vi "PRAMMS-DataString2Image.vi"(7 "ImageData":u8[](array[numeric])) -> (1 "Width":u16, 2 "Height":u16, 3 "BitPerPixel":u32, 8 "Image":u16[][](array[numeric]), 12 "TimeStamp?":u64, 13 "ImageID":u32, 14 "ImageFrameRate":dbl format="%.2f")   [LabVIEW 2019]
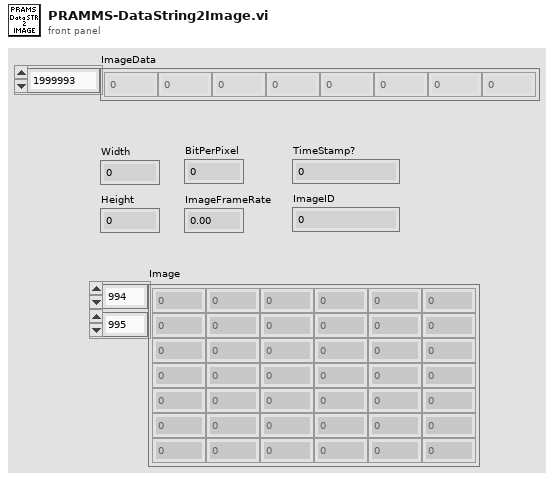
[diagram p1: front panel]
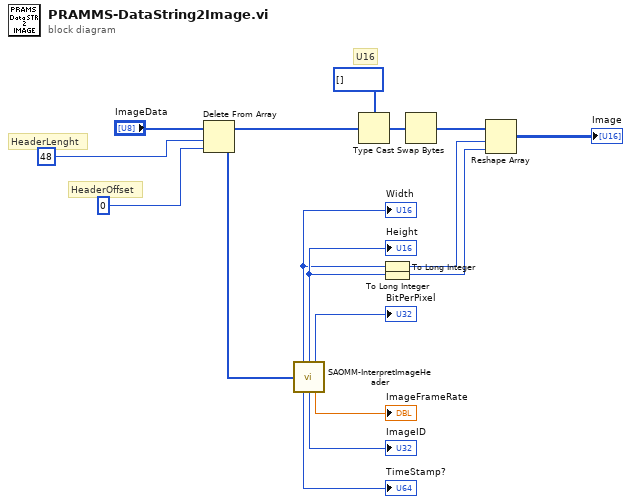
[diagram p0: block diagram]
diagram:
  # "HeaderOffset"
  # "HeaderLenght"
  # "U16"
  n1 = Delete From Array(array="ImageData", length=48 ("index"), index=0) -> (deleted portion=w13:u8[], array with subset deleted=w17:u8[])
  n2 = call "SAOMM-InterpretImageHeader.vi"("ImageHeader"=w13) -> ("ImageWidth"=w6:u16, "ImageHeight"=w7:u16, "BitPerPixel"=→"BitPerPixel":u32, "TimeStamp?"=→"TimeStamp?":u64, "ImageID"=→"ImageID":u32, "ImageFrameRate"=→"ImageFrameRate":dbl)  [unwired: 9 in]
  "Width" <- w6
  "Height" <- w7
  n3 = Type Cast(type=u16[] [], x=w17) -> (*(type *) &x=w12:u16[])
  n4 = To Long Integer(number=w6) -> (32bit integer=w9:i32)
  n5 = To Long Integer(number=w7) -> (32bit integer=w8:i32)
  n6 = Swap Bytes(anything=w12) -> (byte swapped=w10:u16[])
  n7 = Reshape Array(w10, w9, w8) -> (→"Image":u16[][])
